vi "EPTx FPGA add-on test2.vi"() -> ()   [LabVIEW 2019]
uses:
  <vilib>/Powertrain Controls/Device Drivers/Engine Position Tracking/EPTx/RevA/FPGA/Controls/EPTxTooth.ctl
  <vilib>/Powertrain Controls/Device Drivers/Engine Position Tracking/EPTx/RevA/FPGA/Controls/EPTxControl.ctl
  <vilib>/Powertrain Controls/Device Drivers/Engine Position Tracking/EPTx/RevA/FPGA/Controls/EPTxSignals.ctl
  <vilib>/Powertrain Controls/Device Drivers/Engine Position Tracking/EPTx/RevA/FPGA/Controls/EPTxSupervisor.ctl
  <vilib>/Powertrain Controls/Device Drivers/Engine Position Tracking/EPTx/RevA/FPGA/Controls/EPTxConfig.ctl
  <vilib>/Powertrain Controls/Device Drivers/Engine Position Tracking/EPTx/RevA/FPGA/Controls/EPTxPatternConfig.ctl
  <vilib>/Powertrain Controls/Device Drivers/Engine Position Tracking/EPTx/RevA/FPGA/Controls/Patterns.ctl
  <vilib>/Powertrain Controls/Device Drivers/Engine Position Tracking/EPTx/RevA/FPGA/Controls/EPTxDebug.ctl
  <vilib>/Powertrain Controls/Device Drivers/Engine Position Tracking/EPTx/RevA/FPGA/Controls/EPTxAAPControl.ctl
  <vilib>/Powertrain Controls/Device Drivers/Engine Position Tracking/EPTx/RevA/FPGA/Controls/EPTxSimulatorConfig.ctl
  <vilib>/Platform/TimedLoop/XDataNode/timing_clust.ctl
  <vilib>/Platform/TimedLoop/XDataNode/nitl_modes.ctl
  <vilib>/Platform/TimedLoop/XDataNode/wakeup.ctl
  <vilib>/rvi/Emulation/niFpgaSctlEmulationGetInTimedLoop.vi
  <vilib>/rvi/Emulation/niFpgaEmulationReportErrorSimple.vi
  <vilib>/rvi/Emulation/niFpgaGetClockAttributes.vi
  <vilib>/rvi/Emulation/niFpgaCriticalErrorInLSC.vi
  <vilib>/rvi/eio/common/nirviEmuTemplateMethod_errors.vi
  <vilib>/Platform/TimedLoop/XDataNode/XDataNode.xnode
  <vilib>/eio/EIONode/EIONode.xnode
  <vilib>/Platform/TimedLoop/XDataNode/XDNodeRunTimeDep.lvlib
  <vilib>/Powertrain Controls/Device Drivers/Engine Position Tracking/EPTx/RevA/FPGA/EPTx - RevA - FPGA.lvlib
panel:
  in  "CylinderSig_1":T1 caption="簇" {"Cylinder1_L_F [CAD]" format="%.11g"; "Cylinder1_L_R [CAD]" format="%.11g"; "Cylinder1_H_F [CAD]" format="%.11g"; "Cylinder1_H_R [CAD]" format="%.11g"}
  in  "EPTxSimulatorConfig":T2
  in  "AAPControl_1str":T3
  out "EPTxDebug":T4
  in  "EPTxPatternConfig":T5 {"Pattern"."Aux 4" format="%#_16g"; "Pattern"."Aux 3" format="%#_16g"; "Pattern"."Aux 2" format="%#_16g"; "Pattern"."Aux 1" format="%#_16g"; "Pattern"."Primary" format="%#_16g"}
  out "Loop":u32
  in  "EPTxConfig":T7
  out "EPTxSupervisor":T8
  out "EPTxSignals":T9
  in  "EPTxControl":T10
  out "EPTxTooth":T11
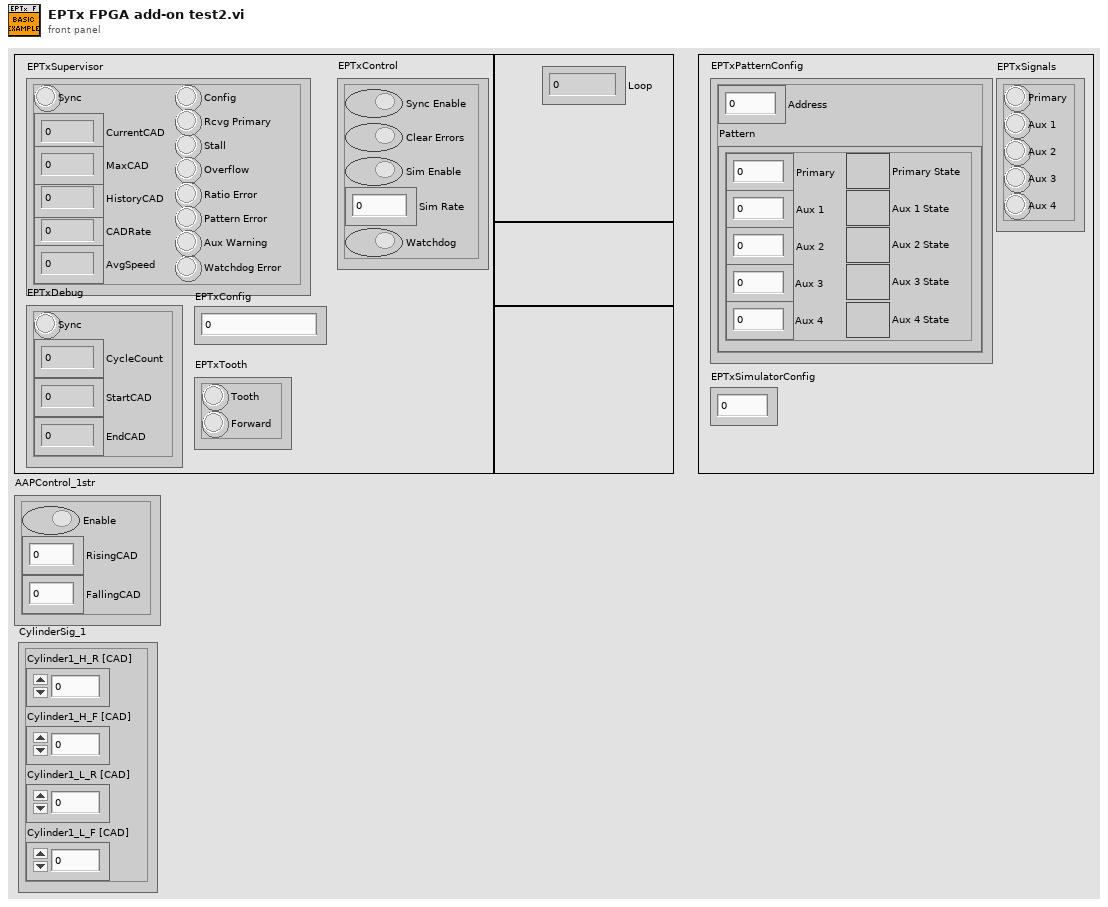
[diagram p1: front panel]
types:
  T1 = cluster{"Cylinder1_H_R [CAD]":fxp<+,18,11>, "Cylinder1_H_F [CAD]":fxp<+,18,11>, "Cylinder1_L_R [CAD]":fxp<+,18,11>, "Cylinder1_L_F [CAD]":fxp<+,18,11>}
  T2 = typedef "EPTx - RevA - FPGA.lvlib/EPTxSimulatorConfig.ctl" = u32
  T3 = typedef "EPTx - RevA - FPGA.lvlib/EPTxAAPControl.ctl" = cluster{"Enable":bool, "RisingCAD":fxp<+,18,11>, "FallingCAD":fxp<+,18,11>}
  T4 = typedef "EPTx - RevA - FPGA.lvlib/EPTxDebug.ctl" = cluster{"Sync":bool, "CycleCount":fxp<+,8,8>, "StartCAD":fxp<+,18,11>, "EndCAD":fxp<+,18,11>}
  T5 = typedef "EPTx - RevA - FPGA.lvlib/EPTxPatternConfig.ctl" = cluster{"Address":fxp<+,14,14>, "Pattern":T6}
  T6 = typedef "EPTx - RevA - FPGA.lvlib/Patterns.ctl" = cluster{"Primary":fxp<+,19,12>, "Primary State":bool, "Aux 1":fxp<+,19,12>, "Aux 1 State":bool, "Aux 2":fxp<+,19,12>, "Aux 2 State":bool, "Aux 3":fxp<+,19,12>, "Aux 3 State":bool, "Aux 4":fxp<+,19,12>, "Aux 4 State":bool}
  T7 = typedef "EPTx - RevA - FPGA.lvlib/EPTxConfig.ctl" = u64
  T8 = typedef "EPTx - RevA - FPGA.lvlib/EPTxSupervisor.ctl" = cluster{"Sync":bool, "CurrentCAD":fxp<+,18,11>, "MaxCAD":fxp<+,11,11>, "HistoryCAD":fxp<+,11,11>, "CADRate":fxp<+,22,8>, "AvgSpeed":fxp<+,17,15>, "Config":bool, "Rcvg Primary":bool, "Stall":bool, "Overflow":bool, "Ratio Error":bool, "Pattern Error":bool, "Aux Warning":bool, "Watchdog Error":bool}
  T9 = typedef "EPTx - RevA - FPGA.lvlib/EPTxSignals.ctl" = cluster{"Primary":bool, "Aux 1":bool, "Aux 2":bool, "Aux 3":bool, "Aux 4":bool}
  T10 = typedef "EPTx - RevA - FPGA.lvlib/EPTxControl.ctl" = cluster{"Sync Enable":bool, "Clear Errors":bool, "Sim Enable":bool, "Sim Rate":fxp<+,24,6>, "Watchdog":bool}
  T11 = typedef "EPTx - RevA - FPGA.lvlib/EPTxTooth.ctl" = cluster{"Tooth":bool, "Forward":bool}
  T12 = typedef "XDNodeRunTimeDep.lvlib/timing_clust.ctl" = cluster{"Expected End [f-1]":u64, "Actual End [f-1]":u64, "Finished Late? [f-1]":bool, "Expected End [i-1]":u64, "Actual End [i-1]":u64, "Finished Late? [i-1]":bool, "Expected Start [i]":u64, "Actual Start [i]":u64, "Expected Start [f]":u64, "Actual Start [f]":u64, "Source Name":string, "Structure Name":string, "Period":i64, "Deadline":i64, "Offset":i64, "Start":i64, "Priority":i32, "Timeout":i32, "Mode":T13, "Wakeup Reason":T14, "Error":errorcluster, "Source Type":string, "Secondary Source Type":string, "Global End Time":u64, "Global Start Time":u64, "Frame Duration":u64, "Iteration Duration":u64, "Assigned CPU":i32, "I/O Scan Engine Mode":u32}
  T13 = typedef "XDNodeRunTimeDep.lvlib/nitl_modes.ctl" = enum32{"No Change", "Process missed periods, maintain original phase", "Discard missed periods, maintain original phase", "Process missed periods, ignore original phase", "Discard missed periods, ignore original phase"}
  T14 = typedef "XDNodeRunTimeDep.lvlib/wakeup.ctl" = enum32{"Normal", "Aborted", "Asynchronous wakeup", "Timing source error", "Timed loop error", "Timeout"}
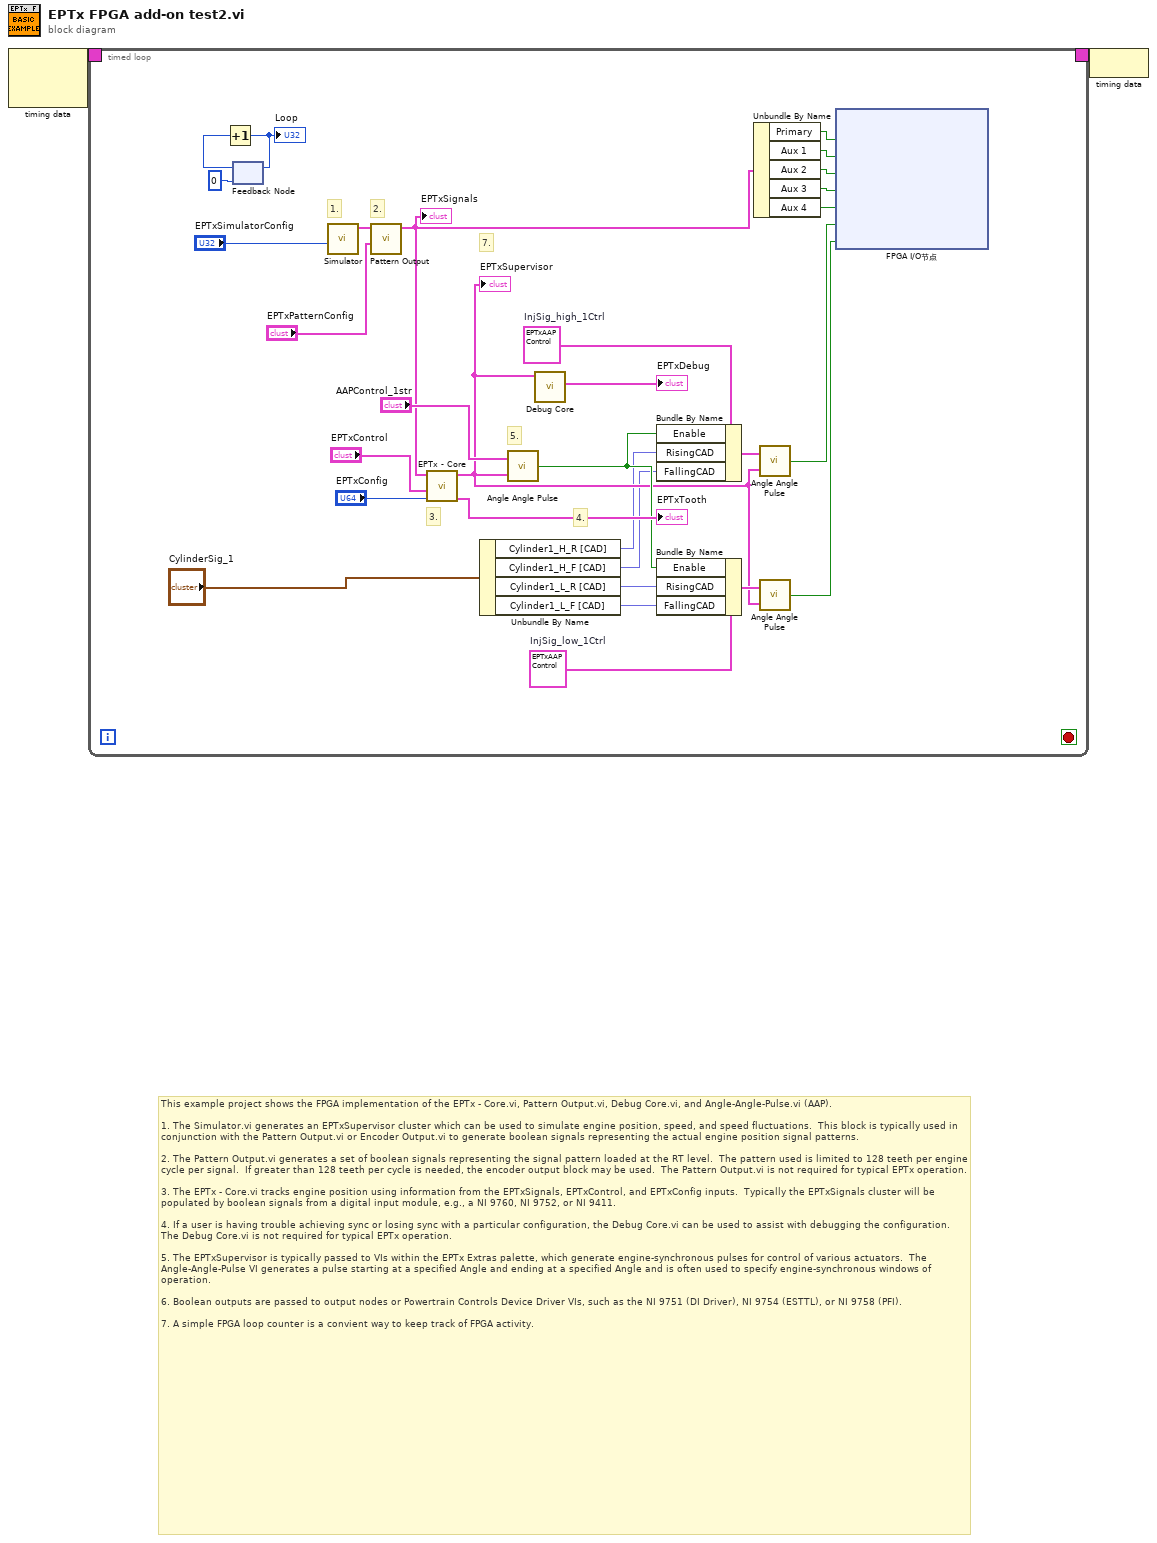
[diagram p0: block diagram]
diagram:
  # "This example project shows the FPGA implementation of the EPTx - Core.vi, Pattern Output.vi, Debug Core.vi, and Angle-Angle-Pulse.vi (AAP).\n\n1. The Simulator.vi generates an EPTxSupervisor cluster which can be used to simulate engine position, speed, and speed fluctuations.  This block is typically used in conjunction with the Pattern Output.vi or Encoder Output.vi to generate boolean signals representing the actual engine position signal patterns.\n\n2. The Pattern Output.vi generates a set of boolean signals representing the signal pattern loaded at the RT level.  The pattern used is limited to 128 teeth per engine cycle per signal.  If greater than 128 teeth per cycle is needed, the encoder output block may be used.  The Pattern Output.vi is not required for typical EPTx operation.\n\n3. The EPTx - Core.vi tracks engine position using information from the EPTxSignals, EPTxControl, and EPTxConfig inputs.  Typically the EPTxSignals cluster will be populated by boolean signals from a digital input module, e.g., a NI 9760, NI 9752, or NI 9411.\n\n4. If a user is having trouble achieving sync or losing sync with a particular configuration, the Debug Core.vi can be used to assist with debugging the configuration.  The Debug Core.vi is not required for typical EPTx operation.\n\n5. The EPTxSupervisor is typically passed to VIs within the EPTx Extras palette, which generate engine-synchronous pulses for control of various actuators.  The Angle-Angle-Pulse VI generates a pulse starting at a specified Angle and ending at a specified Angle and is often used to specify engine-synchronous windows of operation.\n\n6. Boolean outputs are passed to output nodes or Powertrain Controls Device Driver VIs, such as the NI 9751 (DI Driver), NI 9754 (ESTTL), or NI 9758 (PFI).\n\n7. A simple FPGA loop counter is a convient way to keep track of FPGA activity."
  n1 = node-c288() -> (w2:T12)  [unwired: 2 in]
  n2 = timed-loop {
    timing: w2 -> [_]
    timing-out: [_] -> w1
    stop <- _ stop-if-true
    w13 = T3 {"Enable"=FALSE, "RisingCAD"=0.0, "FallingCAD"=0.0}  # InjSig_low_1Ctrl
    w14 = T3 {"Enable"=FALSE, "RisingCAD"=0.0, "FallingCAD"=0.0}  # InjSig_high_1Ctrl
    # "1."
    # "7."
    # "5."
    # "4."
    # "3."
    # "2."
    n3 = feedback #1(u32 0) -> (w29:u32)
    n4 = Increment(x=w29) -> (x+1=w30:u32)
    "Loop" <- w30
    n5 = feedback-in #1(w30) -> ()
    n6 = call <vilib>:"Simulator.vi"("EPTxSimulatorConfig"="EPTxSimulatorConfig") -> ("EPTxSupervisor"=w24:T8)  [unwired: 10 in]
    n7 = call <vilib>:"Pattern Output.vi"("EPTxPatternConfig"="EPTxPatternConfig", "EPTxSupervisor"=w24) -> ("PatternOutput"=w21:T9)  [unwired: 9 in]
    "EPTxSignals" <- w21
    n8 = call <vilib>:"EPTx - Core.vi"("EPTxConfig"="EPTxConfig", "EPTxControl"="EPTxControl", "EPTxSignals"=w21) -> ("EPTxTooth"=→"EPTxTooth":T11, "EPTxSupervisor"=w10:T8)  [unwired: 7 in]
    "EPTxSupervisor" <- w10
    n9 = Unbundle By Name("CylinderSig_1") -> ("Cylinder1_H_R [CAD]"=w8:fxp<+,18,11>, "Cylinder1_H_F [CAD]"=w7:fxp<+,18,11>, "Cylinder1_L_R [CAD]"=w6:fxp<+,18,11>, "Cylinder1_L_F [CAD]"=w5:fxp<+,18,11>)
    n10 = call <vilib>:"Angle Angle Pulse.vi"("EPTxSupervisor"=w10, "AAPControl"="AAPControl_1str") -> ("AAP"=w11:bool)
    n11 = call <vilib>:"Debug Core.vi"("EPTxSupervisor"=w10) -> ("EPTxDebug"=→"EPTxDebug":T4)  [unwired: 10 in]
    n12 = Bundle By Name(cluster=w14, "Enable"=w11, "RisingCAD"=w8, "FallingCAD"=w7) -> (w15:T3)
    n13 = Bundle By Name(cluster=w13, "Enable"=w11, "RisingCAD"=w6, "FallingCAD"=w5) -> (w12:T3)
    n14 = Unbundle By Name(w21) -> ("Primary"=w20:bool, "Aux 1"=w19:bool, "Aux 2"=w18:bool, "Aux 3"=w17:bool, "Aux 4"=w16:bool)
    n15 = call <vilib>:"Angle Angle Pulse.vi"("EPTxSupervisor"=w10, "AAPControl"=w15) -> ("AAP"=w4:bool)
    n16 = call <vilib>:"Angle Angle Pulse.vi"("EPTxSupervisor"=w10, "AAPControl"=w12) -> ("AAP"=w3:bool)
    n17 = xnode "FPGA I/O节点"("Connector0/DIO4"=w20, "Connector0/DIO5"=w19, "Connector0/DIO6"=w18, "Connector0/DIO7"=w17, "Connector0/DIO8"=w16, "Connector0/DIO9"=w4, "Connector0/DIO10"=w3) -> ()  [unwired: 7 in, 7 out]
  }
  n18 = node-c288(w1) -> ()
